vi "AC_6011_DA.vi"(1 "DAData":i32, 2 "DAch":i32, 3 "idd(out)":u32, 4 "hDevice":u32 format="%x") -> (0 "hDevice(out)":i32 format="%x")   [LabVIEW 2015]
uses:
  acpci.dll
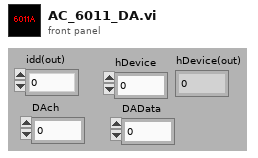
[diagram p1: front panel]
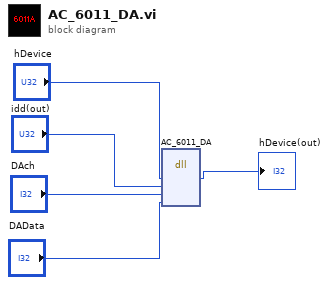
[diagram p0: block diagram]
diagram:
  n1 = dll-call lib="PTH2|abs F2.技术库labviewVI小程序:基于Labview的直流伺服电机位置控制系统设计\t源程序\tACPCI.DLL" fn="AC_6011_DA"("hDevice"="hDevice", "idd"="idd(out)", "DAch"="DAch", "DAData"="DAData") -> ("hDevice"=→"hDevice(out)":u32)  [unwired: 7 in, 2 out]
